vi "SubData2.vi"() -> ()   [LabVIEW 2013]
uses:
  <vilib>/Utility/file.llb/Read From Spreadsheet File (DBL).vi
  <vilib>/Analysis/NI_AALPro.lvlib
panel:
  out "Peak Area Data (V-MHz)":dbl=0.017325289993986456 format="%_3g"
  out "File name 2":string="C:\\Documents and Settings\\Patrick McGaughey\\Desktop\\rssmt\\NMRback.txt"
  out "Residual (V)":dbl=0.000362041158358267 format="%#_3g"
  in  "# of sweeps":i32=500
  out "Spectrum #":i32=499
  out "Chars":i32=640716
  out "Fmin":dbl=212.8 format="%#_13g"
  out "Fmax":dbl=213.2 format="%#_13g"
  out "# Data points":i32=81
  out "Peak Area Fit (V-MHz)":dbl=0.01700494840606724 format="%_3g"
  in  "DC Offset (V)":dbl=0.42 format="%_4g"
  out "RMS Fit Error (V)":dbl=0.005108036034523388 format="%#_2g"
  in  "Start sigma (V)":dbl=0.01 format="%#_13g"
  out "FWHM (MHz)":dbl=0.06647947720746274 format="%#_3g"
  out "Center Freq (MHz)":dbl=213.00722157580975
  out "Amplitude (V)":dbl=0.23986990519803122 format="%_3g"
  out "NMR Thermal Equilibrium Graph + Fit":cluster{cluster{dbl, "Numeric":dbl}[]}[](graph)=[{[{212.8, "Numeric"=5.350526548003441e-13}, {212.805, "Numeric"=1.922601879686162e-12}, {212.81, "Numeric"=6.695995756572205e-12}, {212.815, "Numeric"=2.260340906885167e-11}, {212.82000000000002, "Numeric"=7.395468434586729e-11}, {212.82500000000002, "Numeric"=2.3452567712900613e-10}, {212.83, "Numeric"=7.208552689788091e-10}, {212.835, "Numeric"=2.1475274499866497e-09}, {212.84, "Numeric"=6.201008664265888e-09}, {212.845, "Numeric"=1.735477231887265e-08}, {212.85000000000002, "Numeric"=4.7076966518011464e-08}, {212.85500000000002, "Numeric"=1.2377444527511223e-07}, {212.86, "Numeric"=3.1541800062832327e-07}, {212.865, "Numeric"=7.790672144223506e-07}, {212.87, "Numeric"=1.865075211210947e-06}, {212.875, "Numeric"=4.327636144824661e-06}, {212.88, "Numeric"=9.732806670762442e-06}, {212.88500000000002, "Numeric"=2.1215751605615442e-05}, {212.89000000000001, "Numeric"=4.48241141189609e-05}, {212.895, "Numeric"=9.17905508486164e-05}, {212.9, "Numeric"=0.00018218692467403657}, {212.905, "Numeric"=0.0003504849724646379}, {212.91, "Numeric"=0.0006535135042702434}, {212.915, "Numeric"=0.0011810620060612364}, {212.92000000000002, "Numeric"=0.002068825207109912}, {212.925, "Numeric"=0.003512431532531306}, {212.93, "Numeric"=0.005779960938374233}, {212.935, "Numeric"=0.009218810915490198}, {212.94, "Numeric"=0.0142514114661939}, {212.945, "Numeric"=0.021353733528172297}, {212.95, "Numeric"=0.031011496661889227}, {212.955, "Numeric"=0.04365204576926799}, {212.96, "Numeric"=0.05955516678048669}, {212.965, "Numeric"=0.07875302714131566}, {212.97, "Numeric"=0.10093645213142498}, {212.975, "Numeric"=0.12538967662073625}, {212.98, "Numeric"=0.1509762024133628}, {212.985, "Numeric"=0.1761928091281378}, {212.99, "Numeric"=0.1992970316474099}, {212.995, "Numeric"=0.21849748816925668}, {213.0, "Numeric"=0.23218012196190335}, {213.005, "Numeric"=0.23913139046809306}, {213.01, "Numeric"=0.23871577049681983}, {213.015, "Numeric"=0.2309716096793565}, {213.02, "Numeric"=0.21660528994680797}, {213.025, "Numeric"=0.196884934008013}, {213.03, "Numeric"=0.1734558206018694}, {213.035, "Numeric"=0.14811472592276792}, {213.04, "Numeric"=0.12258591371981398}, {213.045, "Numeric"=0.09833675333463586}, {213.05, "Numeric"=0.07645821075172246}, {213.055, "Numeric"=0.05761895313772516}, {213.06, "Numeric"=0.042086185413200215}, {213.065, "Numeric"=0.029795229348730475}, {213.07, "Numeric"=0.020444988434563188}, {213.075, "Numeric"=0.013597528368265268}, {213.07999999999998, "Numeric"=0.00876528508411346}, {213.085, "Numeric"=0.005476525142322461}, {213.09, "Numeric"=0.0033164777940856744}, {213.095, "Numeric"=0.0019466239824201816}, {213.1, "Numeric"=0.001107439508824899}, {213.105, "Numeric"=0.000610647980024315}, {213.10999999999999, "Numeric"=0.00032635840672995165}, {213.11499999999998, "Numeric"=0.00016905641361237853}, {213.12, "Numeric"=8.487923695789037e-05}, {213.125, "Numeric"=4.130515438555971e-05}, {213.13, "Numeric"=1.9482289865373428e-05}, {213.135, "Numeric"=8.906533780946226e-06}, {213.14, "Numeric"=3.94648454239353e-06}, {213.14499999999998, "Numeric"=1.69490382823417e-06}, {213.14999999999998, "Numeric"=7.055254477154328e-07}, {213.155, "Numeric"=2.84651366659758e-07}, {213.16, "Numeric"=1.1131324190760306e-07}, {213.165, "Numeric"=4.2190372268430824e-08}, {213.17, "Numeric"=1.5499327368103473e-08}, {213.17499999999998, "Numeric"=5.518808354094702e-09}, {213.17999999999998, "Numeric"=1.9046305350072406e-09}, {213.185, "Numeric"=6.371022518946845e-10}, {213.19, "Numeric"=2.065572797328865e-10}, {213.195, "Numeric"=6.490898809754293e-11}, {213.2, "Numeric"=1.976979380918416e-11}]}, {[{212.8, "Numeric"=0.0009524809613886147}, {212.805, "Numeric"=-0.0013545400820829973}, {212.81, "Numeric"=-0.0004320821710246157}, {212.815, "Numeric"=-0.0006217645516615304}, {212.82000000000002, "Numeric"=-0.00204053314008636}, {212.82500000000002, "Numeric"=-0.0014856505351262294}, {212.83, "Numeric"=-0.001531437594602143}, {212.835, "Numeric"=-0.0014040211856031159}, {212.84, "Numeric"=-0.0022403508903871537}, {212.845, "Numeric"=-0.001008341002067002}, {212.85000000000002, "Numeric"=-0.001172253489790096}, {212.85500000000002, "Numeric"=-0.0026446438145235796}, {212.86, "Numeric"=-0.002580024836836758}, {212.865, "Numeric"=0.0001968912734680745}, {212.87, "Numeric"=-0.0017855865180964143}, {212.875, "Numeric"=-0.001559418818509528}, {212.88, "Numeric"=-0.0009337949309199642}, {212.88500000000002, "Numeric"=-0.0041159301804600925}, {212.89000000000001, "Numeric"=-0.00014423894377558016}, {212.895, "Numeric"=-0.0016478196089629393}, {212.9, "Numeric"=-0.001732956463751037}, {212.905, "Numeric"=-0.0013487765556307173}, {212.91, "Numeric"=-0.0006146577928481511}, {212.915, "Numeric"=0.0006137165510511358}, {212.92000000000002, "Numeric"=-0.00246046648967112}, {212.925, "Numeric"=0.00020888610274218136}, {212.93, "Numeric"=-0.003848237491478627}, {212.935, "Numeric"=-0.002449048390439447}, {212.94, "Numeric"=-0.006311992628519216}, {212.945, "Numeric"=-0.008164918898915801}, {212.95, "Numeric"=-0.010267013695960867}, {212.955, "Numeric"=-0.011274772222169768}, {212.96, "Numeric"=-0.009937138724371778}, {212.965, "Numeric"=-0.004833212512056098}, {212.97, "Numeric"=0.0022431450629633804}, {212.975, "Numeric"=0.009001380493490009}, {212.98, "Numeric"=0.014545901795050364}, {212.985, "Numeric"=0.013316911312749298}, {212.99, "Numeric"=0.01139955552694245}, {212.995, "Numeric"=0.0059636851774385}, {213.0, "Numeric"=0.0020635093006217083}, {213.005, "Numeric"=0.0007385143415243152}, {213.01, "Numeric"=0.00012793290998973738}, {213.015, "Numeric"=0.0043630907214388765}, {213.02, "Numeric"=0.007166754141372805}, {213.025, "Numeric"=0.011996129118242174}, {213.03, "Numeric"=0.013474453947229372}, {213.035, "Numeric"=0.01017084822552715}, {213.04, "Numeric"=0.005446272652927481}, {213.045, "Numeric"=-0.003190868565103196}, {213.05, "Numeric"=-0.006442250831876682}, {213.055, "Numeric"=-0.008701581394234496}, {213.06, "Numeric"=-0.006973179401174803}, {213.065, "Numeric"=-0.005758132154342935}, {213.07, "Numeric"=-0.0022742850277534168}, {213.075, "Numeric"=0.0005906129142932222}, {213.07999999999998, "Numeric"=0.0010888271403259727}, {213.085, "Numeric"=0.005205509927822636}, {213.09, "Numeric"=0.004034975111728114}, {213.095, "Numeric"=0.004459284835214398}, {213.1, "Numeric"=0.004705774920029186}, {213.105, "Numeric"=0.0034071145450191367}, {213.10999999999999, "Numeric"=0.003625994298671098}, {213.11499999999998, "Numeric"=0.0024208684360740268}, {213.12, "Numeric"=0.004037529580680507}, {213.125, "Numeric"=0.001378369194311858}, {213.13, "Numeric"=0.002405678030772703}, {213.135, "Numeric"=0.002350232744769696}, {213.14, "Numeric"=0.002299692794004842}, {213.14499999999998, "Numeric"=0.001810137761489015}, {213.14999999999998, "Numeric"=0.0005825349554971614}, {213.155, "Numeric"=0.0014107243666702661}, {213.16, "Numeric"=-0.0002707165236653581}, {213.165, "Numeric"=0.0011893175290603865}, {213.17, "Numeric"=-0.000715761190720014}, {213.17499999999998, "Numeric"=0.00020213776775108218}, {213.17999999999998, "Numeric"=-2.0942894176702704e-06}, {213.185, "Numeric"=-0.0025334779918098106}, {213.19, "Numeric"=-0.000593790386919896}, {213.195, "Numeric"=-0.0014416614677203825}, {213.2, "Numeric"=-0.0010266192582565014}]}, {[{212.8, "Numeric"=0.0009524809619236674}, {212.805, "Numeric"=-0.0013545400801603955}, {212.81, "Numeric"=-0.00043208216432861997}, {212.815, "Numeric"=-0.0006217645290581212}, {212.82000000000002, "Numeric"=-0.0020405330661316754}, {212.82500000000002, "Numeric"=-0.001485650300600552}, {212.83, "Numeric"=-0.0015314368737468738}, {212.835, "Numeric"=-0.001404019038075666}, {212.84, "Numeric"=-0.002240344689378489}, {212.845, "Numeric"=-0.0010083236472946831}, {212.85000000000002, "Numeric"=-0.001172206412823578}, {212.85500000000002, "Numeric"=-0.0026445200400783044}, {212.86, "Numeric"=-0.0025797094188361297}, {212.865, "Numeric"=0.00019767034068249683}, {212.87, "Numeric"=-0.0017837214428852034}, {212.875, "Numeric"=-0.0015550911823647034}, {212.88, "Numeric"=-0.0009240621242492017}, {212.88500000000002, "Numeric"=-0.004094714428854476}, {212.89000000000001, "Numeric"=-9.941482965661928e-05}, {212.895, "Numeric"=-0.001556029058114323}, {212.9, "Numeric"=-0.0015507695390770005}, {212.905, "Numeric"=-0.0009982915831660793}, {212.91, "Numeric"=3.885571142209238e-05}, {212.915, "Numeric"=0.0017947785571123722}, {212.92000000000002, "Numeric"=-0.0003916412825612082}, {212.925, "Numeric"=0.003721317635273487}, {212.93, "Numeric"=0.0019317234468956069}, {212.935, "Numeric"=0.006769762525050752}, {212.94, "Numeric"=0.007939418837674685}, {212.945, "Numeric"=0.013188814629256496}, {212.95, "Numeric"=0.02074448296592836}, {212.955, "Numeric"=0.03237727354709822}, {212.96, "Numeric"=0.04961802805611491}, {212.965, "Numeric"=0.07391981462925955}, {212.97, "Numeric"=0.10317959719438836}, {212.975, "Numeric"=0.13439105711422628}, {212.98, "Numeric"=0.16552210420841315}, {212.985, "Numeric"=0.1895097204408871}, {212.99, "Numeric"=0.21069658717435233}, {212.995, "Numeric"=0.2244611733466952}, {213.0, "Numeric"=0.23424363126252506}, {213.005, "Numeric"=0.2398699048096174}, {213.01, "Numeric"=0.23884370340680955}, {213.015, "Numeric"=0.23533470040079538}, {213.02, "Numeric"=0.22377204408818077}, {213.025, "Numeric"=0.20888106312625515}, {213.03, "Numeric"=0.18693027454909877}, {213.035, "Numeric"=0.15828557414829508}, {213.04, "Numeric"=0.12803218637274147}, {213.045, "Numeric"=0.09514588476953266}, {213.05, "Numeric"=0.07001595991984577}, {213.055, "Numeric"=0.048917371743490666}, {213.06, "Numeric"=0.03511300601202542}, {213.065, "Numeric"=0.024037097194387538}, {213.07, "Numeric"=0.01817070340680977}, {213.075, "Numeric"=0.014188141282558492}, {213.07999999999998, "Numeric"=0.009854112224439434}, {213.085, "Numeric"=0.010682035070145098}, {213.09, "Numeric"=0.007351452905813788}, {213.095, "Numeric"=0.006405908817634579}, {213.1, "Numeric"=0.005813214428854085}, {213.105, "Numeric"=0.004017762525043452}, {213.10999999999999, "Numeric"=0.003952352705401049}, {213.11499999999998, "Numeric"=0.0025899248496864054}, {213.12, "Numeric"=0.004122408817638396}, {213.125, "Numeric"=0.0014196743486974178}, {213.13, "Numeric"=0.002425160320638077}, {213.135, "Numeric"=0.002359139278550642}, {213.14, "Numeric"=0.0023036392785472353}, {213.14499999999998, "Numeric"=0.0018118326653172492}, {213.14999999999998, "Numeric"=0.0005832404809448769}, {213.155, "Numeric"=0.0014110090180369259}, {213.16, "Numeric"=-0.00027060521042345046}, {213.165, "Numeric"=0.001189359719432655}, {213.17, "Numeric"=-0.0007157456913926459}, {213.17499999999998, "Numeric"=0.00020214328655943626}, {213.17999999999998, "Numeric"=-2.092384787135263e-06}, {213.185, "Numeric"=-0.0025334773547075586}, {213.19, "Numeric"=-0.0005937901803626163}, {213.195, "Numeric"=-0.0014416614028113944}, {213.2, "Numeric"=-0.0010266192384867075}]}]
  out "File size (bytes)":i32=1284000
  out "File name":string="C:\\Documents and Settings\\Patrick McGaughey\\Desktop\\rssmt\\NMR3489061581.xls"
  # "Gaussian Fit Results"
  # "Integration Results"
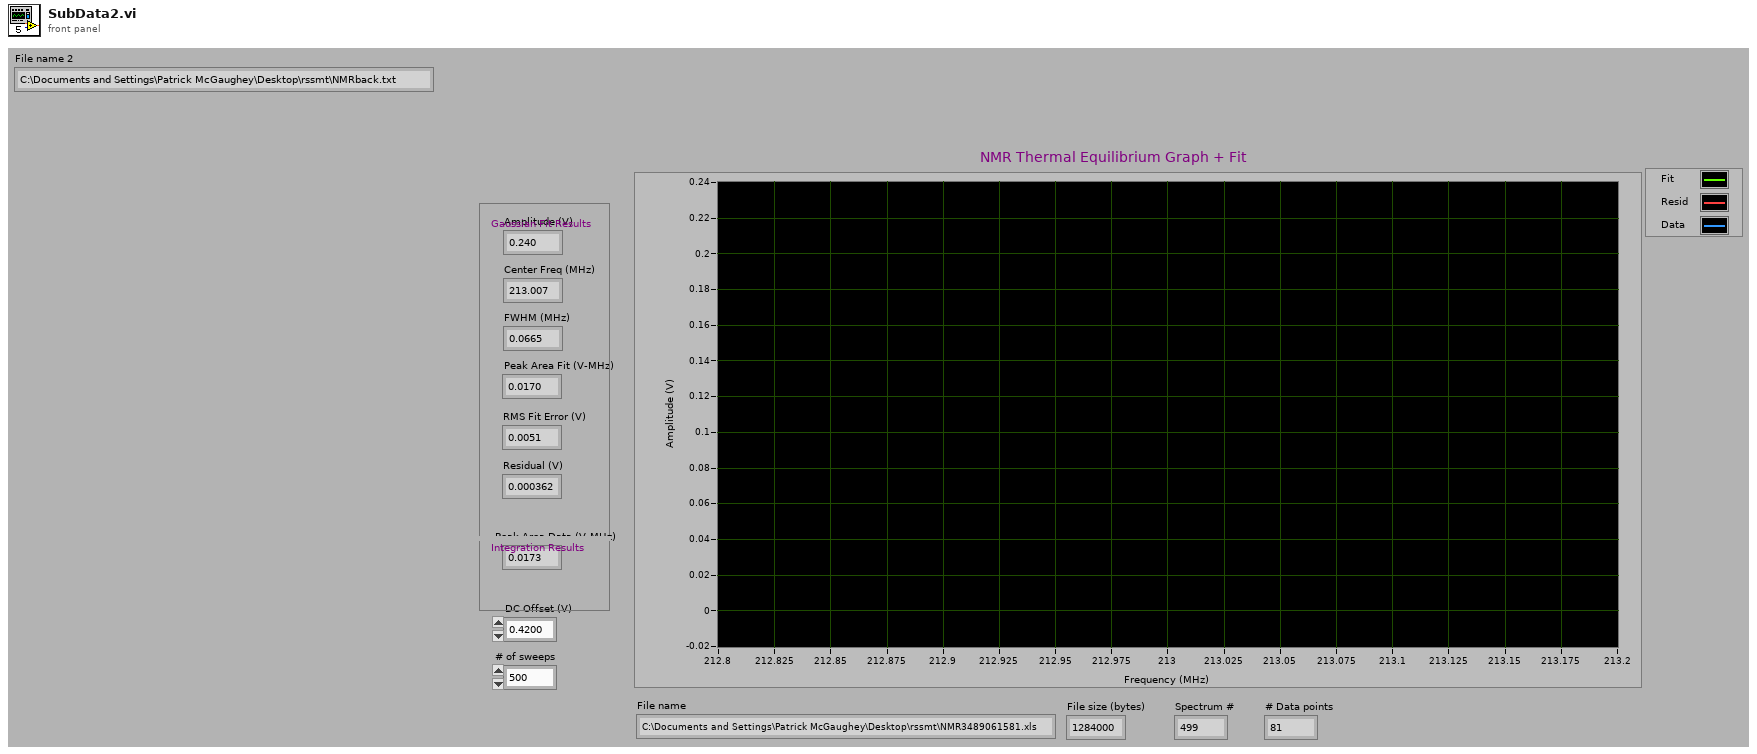
[diagram p1: front panel]
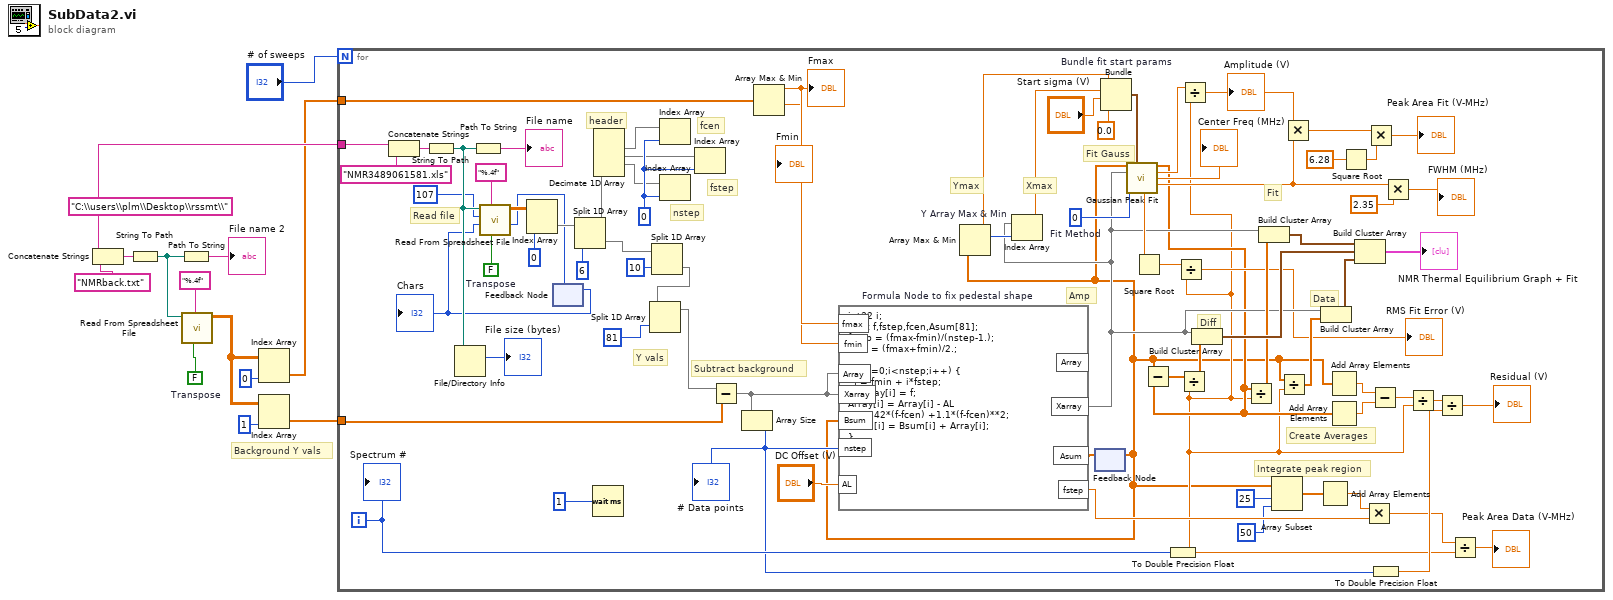
[diagram p0: block diagram]
diagram:
  w9 = FALSE  # Transpose
  w2 = "C:\\users\\plm\\Desktop\\rssmt\\"
  # "Background Y vals"
  n1 = Concatenate Strings "Concatenate Strings"(w2, "NMRback.txt") -> (w12:string)
  n2 = String To Path(string=w12) -> (path=w8:path)
  n3 = Path To String(path=w8) -> (string=→"File name 2":string)
  n4 = call-poly <vilib>:"Read From Spreadsheet File.vi"("transpose (no:F)"=w9, "format (%.3f)"="%.4f", "file path (dialog if empty)"=w8) -> ("all rows"=w7:dbl[][])  [unwired: 4 in, 4 out]
  n5 = Index Array "Index Array"(array=w7, index (col)=0) -> (element=w1:dbl[])  [unwired: 1 in]
  n6 = Index Array(array=w7, index (col)=1) -> (element=w3:dbl[])  [unwired: 1 in]
  n7 = for {
    N: "# of sweeps" -> [_]
    tunnel: w3 -> [w25]
    tunnel: w2 -> [w31]
    tunnel: w1 -> [w29]
    i -> [w53]
    w66 = 0
    w83 = 0  # Fit Method
    w90 = FALSE  # Transpose
    # "Integrate peak region"
    # "Create Averages"
    # "Diff"
    # "Fit"
    # "Data"
    # "fcen"
    # "Fit Gauss"
    # "Read file"
    # "header"
    # "nstep"
    # "fstep"
    # "Amp"
    # "Subtract background"
    # "Ymax"
    # "Xmax"
    # "Y vals"
    n8 = Concatenate Strings "Concatenate Strings"(w31, "NMR3489061581.xls") -> (w93:string)
    n9 = String To Path(string=w93) -> (path=w89:path)
    n10 = File/Directory Info(path=w89) -> (size=→"File size (bytes)":i64)  [unwired: 1 in, 6 out]
    n11 = Path To String(path=w89) -> (string=→"File name":string)
    n12 = feedback #1() -> (w59:i32)  [unwired: 1 in]
    "Chars" <- w59
    n13 = call-poly <vilib>:"Read From Spreadsheet File.vi"("transpose (no:F)"=w90, "format (%.3f)"="%.4f", "start of read offset (chars.:0)"=w59, "number of rows (all:-1)"=107, "file path (dialog if empty)"=w89) -> ("mark after read (chars.)"=w60:i32, "all rows"=w70:dbl[][])  [unwired: 2 in, 3 out]
    n14 = Index Array "Index Array"(array=w70, index (col)=0) -> (element=w68:dbl[])  [unwired: 1 in]
    n15 = feedback-in #1(w60) -> ()
    n16 = Split 1D Array(array=w68, index=6) -> (first subarray=w71:dbl[], second subarray=w52:dbl[])
    n17 = Wait (ms)(milliseconds to wait=1) -> ()  [unwired: 1 out]
    n18 = Decimate 1D Array(w71) -> (w67:dbl[], w65:dbl[], w64:dbl[])  [unwired: 3 out]
    n19 = Split 1D Array(array=w52, index=10) -> (second subarray=w50:dbl[])  [unwired: 1 out]
    n20 = Split 1D Array(array=w50, index=81) -> (first subarray=w33:dbl[])  [unwired: 1 out]
    n21 = Index Array "Index Array"(array=w67, index=w66) -> ()  [unwired: 1 out]
    n22 = Index Array(array=w64, index=w66) -> ()  [unwired: 1 out]
    n23 = Index Array(array=w65, index=w66) -> ()  [unwired: 1 out]
    n24 = Subtract(x=w33, y=w25) -> (x-y=w32:dbl[])
    n25 = Array Size(array=w32) -> (size(s)=w26:i32)
    "# Data points" <- w26
    n26 = Array Max & Min(array=w29) -> (max value=w28:dbl, min value=w27:dbl)  [unwired: 2 out]
    "Fmax" <- w28
    "Fmin" <- w27
    n27 = feedback #2() -> (w16:dbl[])  [unwired: 1 in]
    n28 = formula code="int32 i;\nfloat f,fstep,fcen,Asum[81];\nfstep = (fmax-fmin)/(nstep-1.);\nfcen = (fmax+fmin)/2.;\n\nfor (i=0;i<nstep;i++) {\n  f = fmin + i*fstep;\n  Xarray[i] = f;\nArray[i] = Array[i] - AL \n   +0.42*(f-fcen) +1.1*(f-fcen)**2;\nAsum[i] = Bsum[i] + Array[i];\n}" "Formula Node to fix pedestal shape"("nstep"=w26, "fmin"=w27, "fmax"=w28, "AL"="DC Offset (V)", "Array"=w32, "Xarray"=w32, "Bsum"=w16) -> ("Xarray"=w44:dbl[], "Asum"=w57:dbl[], "fstep"=w22:dbl)  [unwired: 1 out]
    n29 = Array Max & Min "Y Array Max & Min"(array=w16) -> (max value=w82:dbl, max index (indices)=w81:i32)  [unwired: 2 out]
    n30 = Index Array "Index Array"(array=w44, index=w81) -> (element=w76:dbl)
    n31 = feedback-in #2(w57) -> ()
    n32 = Bundle "Bundle fit start params"(w82, w76, "Start sigma (V)"="Start sigma (V)", 0.0) -> (w86:cluster{dbl, dbl, "Start sigma (V)":dbl, dbl})  [unwired: 1 in]
    n33 = call <vilib>:"Gaussian Peak Fit.vi"("Y"=w16, "initial guess"=w86, "X"=w44, "method"=w83) -> ("Best Gaussian Fit"=w39:dbl[], "amplitude"=w46:dbl, "center"=→"Center Freq (MHz)":dbl, "standard deviation"=w75:dbl, "residue"=w77:dbl)  [unwired: 5 in, 2 out]
    n34 = Square Root(x=w77) -> (sqrt(x)=w41:dbl)
    n35 = Subtract(x=w16, y=w39) -> (x-y=w55:dbl[])
    n36 = To Double Precision Float(number=w53) -> (double precision float=w20:dbl)
    n37 = Divide(x=w41, y=w20) -> (x/y=→"RMS Fit Error (V)":dbl)
    n38 = Divide(x=w55, y=w20) -> (x/y=w54:dbl[])
    n39 = Divide(x=w46, y=w20) -> (x/y=w45:dbl)
    "Amplitude (V)" <- w45
    n40 = Build Cluster Array ("Index & Bundle Cluster Array")(w44, w54) -> (w56:cluster{dbl, dbl}[])
    n41 = Divide(x=w39, y=w20) -> (x/y=w47:dbl[])
    n42 = Build Cluster Array ("Index & Bundle Cluster Array")(w44, w47) -> (w63:cluster{dbl, dbl}[])
    n43 = Array Subset(array=w16, index=25, length=50) -> (w17:dbl[])
    n44 = Divide(x=w16, y=w20) -> (x/y=w42:dbl[])
    n45 = Multiply(x=w45, y=w75) -> (x*y=w78:dbl)
    n46 = Add Array Elements(numeric array=w17) -> (sum=w18:dbl)
    n47 = Build Cluster Array ("Index & Bundle Cluster Array")(w44, w42) -> (w43:cluster{dbl, dbl}[])
    n48 = Add Array Elements(numeric array=w16) -> (sum=w23:dbl)
    n49 = Add Array Elements(numeric array=w39) -> (sum=w38:dbl)
    n50 = Square Root(x=6.28) -> (sqrt(x)=w79:dbl)
    n51 = Build Cluster Array "Build Cluster Array"(w63, w56, w43) -> (→"NMR Thermal Equilibrium Graph + Fit":cluster{cluster{dbl, dbl}[]}[])
    n52 = Multiply(x=w18, y=w22) -> (x*y=w21:dbl)
    n53 = Multiply(x=w78, y=w79) -> (x*y=→"Peak Area Fit (V-MHz)":dbl)
    n54 = Subtract(x=w23, y=w38) -> (x-y=w37:dbl)
    n55 = To Double Precision Float(number=w26) -> (double precision float=w34:dbl)
    n56 = Multiply(x=w75, y=2.35) -> (x*y=→"FWHM (MHz)":dbl)
    n57 = Divide(x=w37, y=w20) -> (x/y=w36:dbl)
    n58 = Divide(x=w36, y=w34) -> (x/y=→"Residual (V)":dbl)
    n59 = Divide(x=w21, y=w20) -> (x/y=→"Peak Area Data (V-MHz)":dbl)
    "Spectrum #" <- w53
  }
